vi "Tetra_Filt.vi"(0 "COMPORT":refnum<visa-resource-name>="COM4", 1 "ADAR-ID":i32(ring) items=["ALL", "ADAR-1", "ADAR-2", "ADAR-3"], 3 "Rev-C(T)":bool=TRUE, 5 "error in (no error)":errorcluster, 6 "RO(t)":bool, 7 "RX/TX":i32(ring)=1 items=["RX", "TX"], 9 "Filt(sel)":i32(ring)=2 items=["OFF", "LOW", "MID", "HIGH"], 11 "Open Ser(t)":bool, 13 "Close Ser(t)":bool) -> (10 "filt(num)":i32, 14 "comport":refnum<visa-resource-name>="COM4", 19 "error out":errorcluster)   [LabVIEW 2018]
panel:
  out "cmd":string
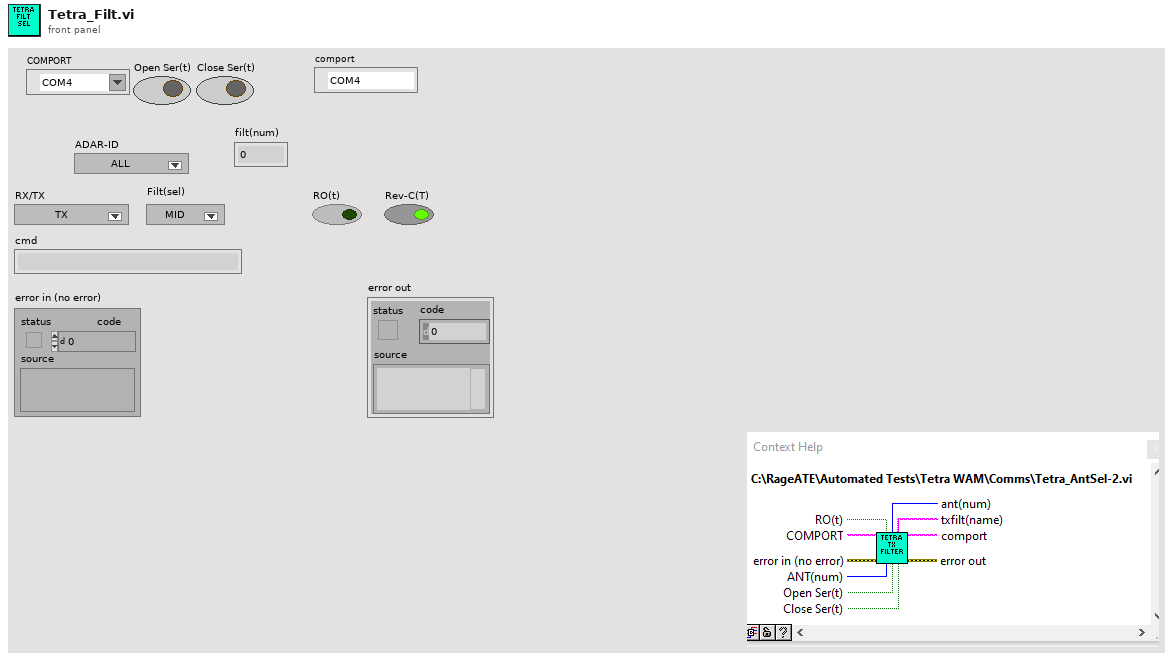
[diagram p1: front panel]
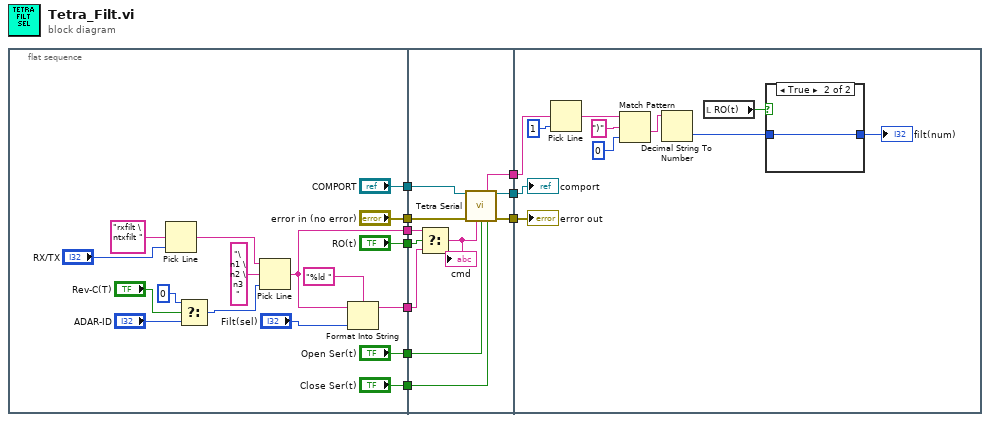
[diagram p0: block diagram]
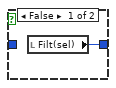
[diagram p2: hidden frame]
diagram:
  n1 = flat-sequence {
    tunnel: ["error in (no error)"] -> w10
    tunnel: ["COMPORT"] -> w9
    tunnel: [w24] -> w8
    tunnel: ["Open Ser(t)"] -> w7
    tunnel: [w16] -> w6
    tunnel: ["Close Ser(t)"] -> w5
    tunnel: ["RO(t)"] -> w2
    tunnel: w10 -> [w38]
    tunnel: w9 -> [w37]
    tunnel: w8 -> [w36]
    tunnel: w7 -> [w35]
    tunnel: w6 -> [w30]
    tunnel: w5 -> [w32]
    tunnel: [w34] -> w4
    tunnel: [w33] -> w3
    tunnel: w2 -> [w29]
    tunnel: [w31] -> w1
    tunnel: w1 -> [w45]
    tunnel: w3 -> [w44]
    tunnel: w4 -> [w43]
    frame #0 {
      n2 = Pick Line(multi-line string="rxfilt \ntxfilt ", line index="RX/TX") -> (output string=w17:string)  [unwired: 1 in]
      n3 = Select(t=0, s="Rev-C(T)", f="ADAR-ID") -> (s? t:f=w11:i32)
      n4 = Pick Line(string ("")=w17, multi-line string="\n1 \n2 \n3 ", line index=w11) -> (output string=w16:string)
      n5 = Format Into String(format string="%ld ", initial string=w16, "Filt(sel)") -> (resulting string=w24:string)  [unwired: 1 in, 1 out]
    }
    frame #1 {
      n6 = Select(t=w30, s=w29, f=w36) -> (s? t:f=w28:string)
      "cmd" <- w28
      n7 = call "Tetra Serial.vi"("COMPORT"=w37, "error in (no error)"=w38, "Command"=w28, "Open Ser(t)"=w35, "Close Ser(t)"=w32) -> ("output"=w31:string, "comport"=w33:refnum<visa-resource-name>, "error out"=w34:errorcluster)  [unwired: 6 in, 2 out]
    }
    frame #2 {
      n8 = Pick Line(multi-line string=w45, line index=1) -> (output string=w49:string)  [unwired: 1 in]
      n9 = Match Pattern(string=w49, regular expression=")", offset (0)=0) -> (after substring=w39:string)  [unwired: 3 out]
      n10 = Decimal String To Number(string=w39) -> (number=w42:i32)  [unwired: 2 in, 1 out]
      n11 = local read "RO(t)"() -> (w40:bool)
      n12 = case shown="True" w40 {
        tunnel: w42 -> [_ w51]
        tunnel: [w50 w51] -> w41
        frame False {
          n13 = local read "Filt(sel)"() -> (w50:i32)
        }
        frame True {
        }
      }
      "filt(num)" <- w41
      "comport" <- w44
      "error out" <- w43
    }
  }
